vi "SH_saveShapelets.vi"(8 "error in (no error)":errorcluster, 9 "Pruning on?":bool, 10 "Indicies":i32[](array[numeric]), 11 "ShapeletClass in":refnum<class "Shapelets Search Brute Force.lvclass">) -> (0 "error out":errorcluster, 3 "ShapeletClass out":refnum<class "Shapelets Search Brute Force.lvclass">)   [LabVIEW 2016, in "Shapelets Search (Brute Force).lvlib" / "Shapelets Search Brute Force.lvclass"]
uses:
  Shapelets Search Brute Force.lvclass
  Shapelets Search Brute Force.lvclass/Shapelets Search Brute Force.ctl
  <vilib>/Analysis/baseanly.llb/Normalize Vector.vi
  <vilib>/Analysis/NI_AALBase.lvlib
panel:
  # "This VI is a part of BCI Design library, http://www.ru-bci.org \nCopyright © 2020, Sotnikov Peter, All rights reserved. License: GNU GPLv3"
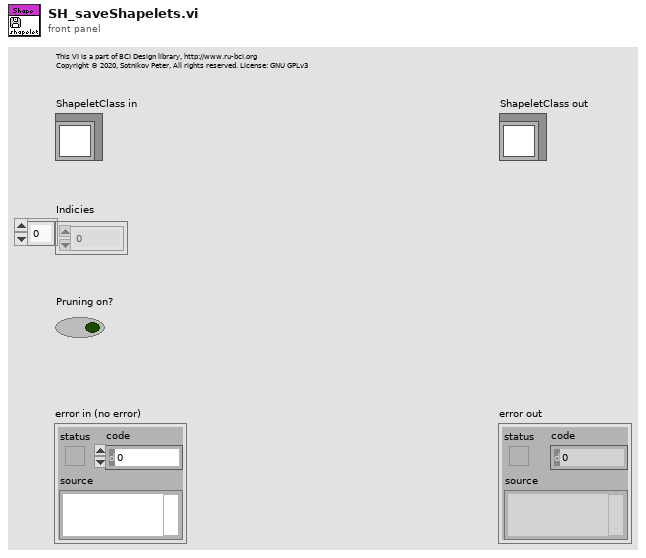
[diagram p1: front panel]
types:
  T1 = enum16{"big-endian, network order", "native, host order", "little-endian"}
  T2 = enum16{"open", "replace", "create", "open or create", "replace or create", "replace or create with confirmation"}
  T3 = cluster{"ClassLabel":string, "FeatureVector":dbl[][]}[]
  T4 = typedef "Shapelets Search (Brute Force).lvlib/SH_Shapelet.ctl" = cluster{"TrialIndex":i32, "Shift (in samples)":i32, "Length (in samples)":i32, "Distances":dbl[], "ClassIndecies":i32[], "Fitness":dbl, "Split Point":dbl}
  T5 = cluster{"ClassLabel":string, "FeatureVector":dbl[][]}
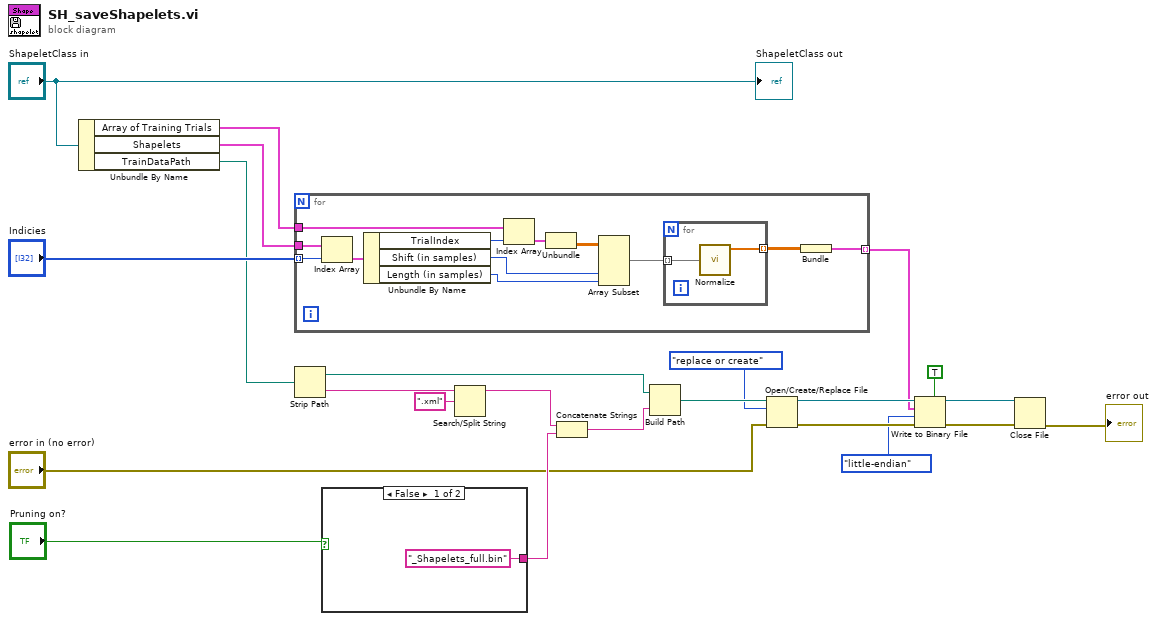
[diagram p0: block diagram]
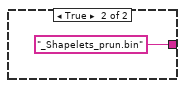
[diagram p2: hidden frame]
diagram:
  n1 = Unbundle By Name("ShapeletClass in") -> ("Array of Training Trials"=w21:T3, "Shapelets"=w20:T4[], "TrainDataPath"=w19:path)
  n2 = for {
    tunnel: "Indicies" -> [w34] mode=indexing
    tunnel: w20 -> [w35]
    tunnel: w21 -> [w31]
    tunnel: [w24] -> w6 mode=indexing
    n3 = Index Array(array=w35, index=w34) -> (element=w33:T4)
    n4 = Unbundle By Name(w33) -> ("TrialIndex"=w32:i32, "Shift (in samples)"=w28:i32, "Length (in samples)"=w27:i32)
    n5 = Index Array(array=w31, index=w32) -> (element=w30:T5)
    n6 = Unbundle(w30) -> ("FeatureVector"=w29:dbl[][])  [unwired: 1 out]
    n7 = Array Subset(array=w29, index (col)=w28, length (col)=w27) -> (w26:dbl[][])  [unwired: 2 in]
    n8 = for {
      tunnel: [w37] -> w25 mode=indexing
      tunnel: w26 -> [w36] mode=indexing
      n9 = call-poly <vilib>:"Normalize.vi"("Vector"=w36) -> ("Normalized Vector"=w37:dbl[])  [unwired: 1 in, 3 out]
    }
    n10 = Bundle("Normalized Vector"=w25) -> (w24:cluster{"Normalized Vector":dbl[][]})  [unwired: 1 in]
  }
  n11 = Strip Path(path=w19) -> (stripped path=w14:path, name=w18:string)
  n12 = case shown="False" "Pruning on?" {
    tunnel: ["_Shapelets_full.bin" ("string") "_Shapelets_prun.bin" ("string")] -> w15
    frame False {
    }
    frame True {
    }
  }
  n13 = Search/Split String(string=w18, search string/char (-)=".xml") -> (substring before match=w16:string)  [unwired: 1 in, 2 out]
  n14 = Concatenate Strings(w16, w15) -> (w13:string)
  n15 = Build Path(base path=w14, name or relative path=w13) -> (appended path=w12:path)
  n16 = Open/Create/Replace File(file path (use dialog)=w12, error in="error in (no error)", operation (0:open)=T2."replace or create") -> (refnum out=w9:refnum<file>, error out=w8:errorcluster)  [unwired: 3 in, 1 out]
  n17 = Write to Binary File(file (use dialog)=w9, data=w6, error in=w8, 5:TRUE ("prepend array or string size? (T)"), 9:T1."little-endian" ("byte order (0:big-endian, network order)")) -> (refnum out=w4:refnum<file>, error out=w3:errorcluster)  [unwired: 1 in, 1 out]
  n18 = Close File(refnum=w4, error in=w3) -> (error out=→"error out":errorcluster)  [unwired: 1 out]
  "ShapeletClass out" <- "ShapeletClass in"
